vi "PID Output Rate Limiter (DBL).vi"(4 "reinitialize? (F)":bool, 6 "dt (s)":dbl=-1.0 format="%.2f", 7 "output rate (EGU/min)":dbl=1.0 format="%.2f", 8 "initial output":dbl format="%.2f", 9 "input (controller output)":dbl format="%.2f") -> (0 "dt out (s)":dbl format="%.3f", 3 "output":dbl format="%.2f")   [LabVIEW 2017, in "NI_PID_pid.lvlib"]
doc: "Limits the rate of change of the controller output. Place this VI immediately after the PID VI in your control application. Use the DBL instance of this VI to implement a single control loop. Use the DBL Array instance to implement parallel multi-loop control."
uses:
  <vilib>/addons/control/pid/NI_PID_pid.lvlib
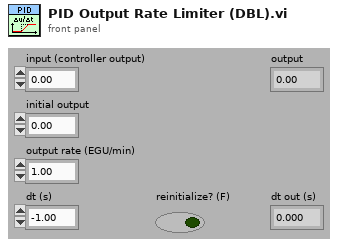
[diagram p1: front panel]
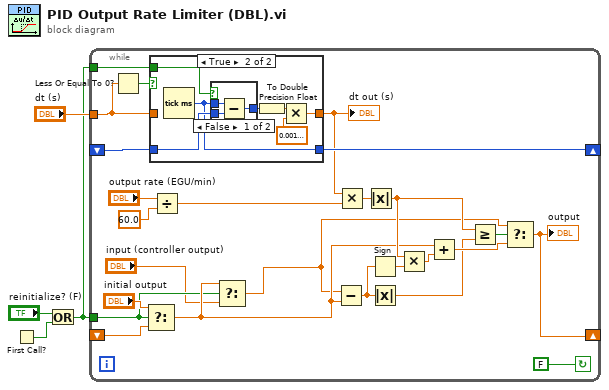
[diagram p0: block diagram]
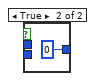
[diagram p3: hidden frame]
diagram:
  n1 = First Call?() -> (First Call?: T/F=w2:bool)
  n2 = Or(x="reinitialize? (F)", y=w2) -> (x .or. y?=w1:bool)
  n3 = while {
    tunnel: w1 -> [w7]
    shift-left: _ -> [w12]
    shift-right: [w11] -> _
    shift-left: _ -> [w16]
    shift-right: [w15] -> _
    tunnel: "dt (s)" -> [w13]
    tunnel: w1 -> [w9]
    stop <- FALSE continue-if-true
    n4 = Less Or Equal To 0?(x=w13) -> (x <= 0?=w14:bool)
    n5 = Select(t="initial output", s=w7, f=w16) -> (s? t:f=w8:dbl)
    n6 = case shown="True" w14 {
      tunnel: [w31 w35] -> w10
      tunnel: w12 -> [w30 w34]
      tunnel: [w30 w33] -> w11
      tunnel: w13 -> [w31 _]
      tunnel: w9 -> [_ w32]
      frame False {
      }
      frame True {
        n7 = Tick Count (ms)() -> (millisecond timer value=w33:u32)
        n8 = case shown="False" w32 {
          tunnel: [w41 u32 0] -> w37
          tunnel: w34 -> [w40 _]
          tunnel: w33 -> [w39 _]
          frame False {
            n9 = Subtract(x=w39, y=w40) -> (x-y=w41:u32)
          }
          frame True {
          }
        }
        n10 = To Double Precision Float(number=w37) -> (double precision float=w36:dbl)
        n11 = Multiply(x=w36, y=0.0010000000474974513) -> (x*y=w35:dbl)
      }
    }
    "dt out (s)" <- w10
    n12 = Divide(x="output rate (EGU/min)", y=60.0) -> (x/y=w28:dbl)
    n13 = Select(t=w8, s=w7, f="input (controller output)") -> (s? t:f=w5:dbl)
    n14 = Subtract(x=w5, y=w8) -> (x-y=w25:dbl)
    n15 = Multiply(x=w10, y=w28) -> (x*y=w27:dbl)
    n16 = Absolute Value(x=w27) -> (abs(x)=w23:dbl)
    n17 = Sign(1:w25) -> (0:w24:dbl)
    n18 = Absolute Value(x=w25) -> (abs(x)=w20:dbl)
    n19 = Multiply(x=w23, y=w24) -> (x*y=w22:dbl)
    n20 = Add(x=w8, y=w22) -> (x+y=w21:dbl)
    n21 = Greater Or Equal?(x=w23, y=w20) -> (x >= y?=w26:bool)
    n22 = Select(t=w5, s=w26, f=w21) -> (s? t:f=w15:dbl)
    "output" <- w15
  }
